vi "AD9959controlMR1_B1.vi"(9 "Enable Master Stepper":bool, 10 "Array":T2(array[cluster])=[{"Enable ASF?"=FALSE, "Channel Frequency (MHz)"=80.0, "ASF"=0.185, "Enable Frequency Sweep"=FALSE, "Sweep Parameters"={"Start Frequency (MHz)"=80.5, "Stop Frequency (MHz)"=89.25, "Rising Step Size (MHz)"=0.04375, "Falling Step Size (MHz)"=0.0, "Falling Step Interval (ms)"=0.01, "Rising Step Interval (ms)"=1.0}, "Rising/Falling"=FALSE}, {"Enable ASF?"=TRUE, "Channel Frequency (MHz)"=110.0, "ASF"=0.185, "Enable Frequency Sweep"=FALSE, "Sweep Parameters"={"Start Frequency (MHz)"=70.0, "Stop Frequency (MHz)"=160.0, "Rising Step Size (MHz)"=0.0006, "Falling Step Size (MHz)"=0.0, "Falling Step Interval (ms)"=0.01, "Rising Step Interval (ms)"=1.0}, "Rising/Falling"=FALSE}, {"Enable ASF?"=FALSE, "Channel Frequency (MHz)"=80.0, "ASF"=0.1, "Enable Frequency Sweep"=FALSE, "Sweep Parameters"={"Start Frequency (MHz)"=80.5, "Stop Frequency (MHz)"=89.25, "Rising Step Size (MHz)"=0.04375, "Falling Step Size (MHz)"=0.0, "Falling Step Interval (ms)"=0.01, "Rising Step Interval (ms)"=1.0}, "Rising/Falling"=FALSE}, {"Enable ASF?"=TRUE, "Channel Frequency (MHz)"=80.0, "ASF"=0.1, "Enable Frequency Sweep"=FALSE, "Sweep Parameters"={"Start Frequency (MHz)"=40.0, "Stop Frequency (MHz)"=115.0, "Rising Step Size (MHz)"=0.0006, "Falling Step Size (MHz)"=0.0, "Falling Step Interval (ms)"=0.01, "Rising Step Interval (ms)"=1.0}, "Rising/Falling"=FALSE}] {"Sweep Parameters"."Rising Step Interval (ms)" min=0.0 max=2.55 step=0.01 format="%.4f"; "Sweep Parameters"."Stop Frequency (MHz)" min=0.0 max=400.0 step=1.0 format="%.6f"; "Sweep Parameters"."Start Frequency (MHz)" min=0.0 max=400.0 step=1.0 format="%.6f"; "Sweep Parameters"."Falling Step Interval (ms)" min=0.0 max=2.55 step=0.01 format="%.2f"; "Sweep Parameters"."Falling Step Size (MHz)" min=0.0 max=400.0 step=0.1 format="%.6f"; "Sweep Parameters"."Rising Step Size (MHz)" min=0.0 max=400.0 step=0.1 format="%.7f"; "ASF" min=0.0 max=1.0 step=0.001 format="%.3f"; "Channel Frequency (MHz)" min=0.0 max=400.0 step=1.0 format="%.6f"}, 11 "VISA Reference":refnum<visa-resource-name>="AD1") -> (2 "Duration array":T1(array[cluster]))   [LabVIEW 2016]
uses:
  <userlib>/configTool/configTool.llb/initConfigGlobal.vi
  <userlib>/configTool/configTool.llb/addProperty(DBL).vi
  <userlib>/configTool/configTool.llb/addProperty(BOOL).vi
  <userlib>/configTool/configTool.llb/saveConfigFile - Text.vi
  <userlib>/configTool/configTool.llb/closeConfig.vi
panel:
  out "Actual Channel Frequencies (MHz)":dbl[](array[numeric]) format="%#_10g"
  out "error out 2":errorcluster
  in  "config file path":path
  in  "Save Config File":bool=TRUE
  in  "Load Config File?":bool=TRUE
  out "System Clock (MHz)":u32
  in  "Multiplier":u32=5
  in  "Reference Clock (MHz)":u32=20
  # "70-160MHz sweep"
  # "40-115MHz sweep"
  # "AD1"
  # "Unused"
  # "AOM3 IntraAction 110 MHz\nProbe 1"
  # "AOM4 Isomet 80 MHz\nProbe 2"
  # "AOM3 Intraction 110 MHz\nCalibration tone"
  # "max 0.115"
  # "max 0.185"
  # "max 0.100"
  # "max 0.185"
  # "Channel 1"
  # "Channel 2"
  # "Channel 3"
  # "Channel 0"
  # "I/O"
  # "Clock"
  # "Profile Pins"
  # "P0 is cut\nP1 is cut\nP2 is cut\nP3 is cut"
  # "Power Down"
  # "Notes:\nMinimum Frequency Step is 0.0931 Hz.\nMinimum ASF Step is 0.001"
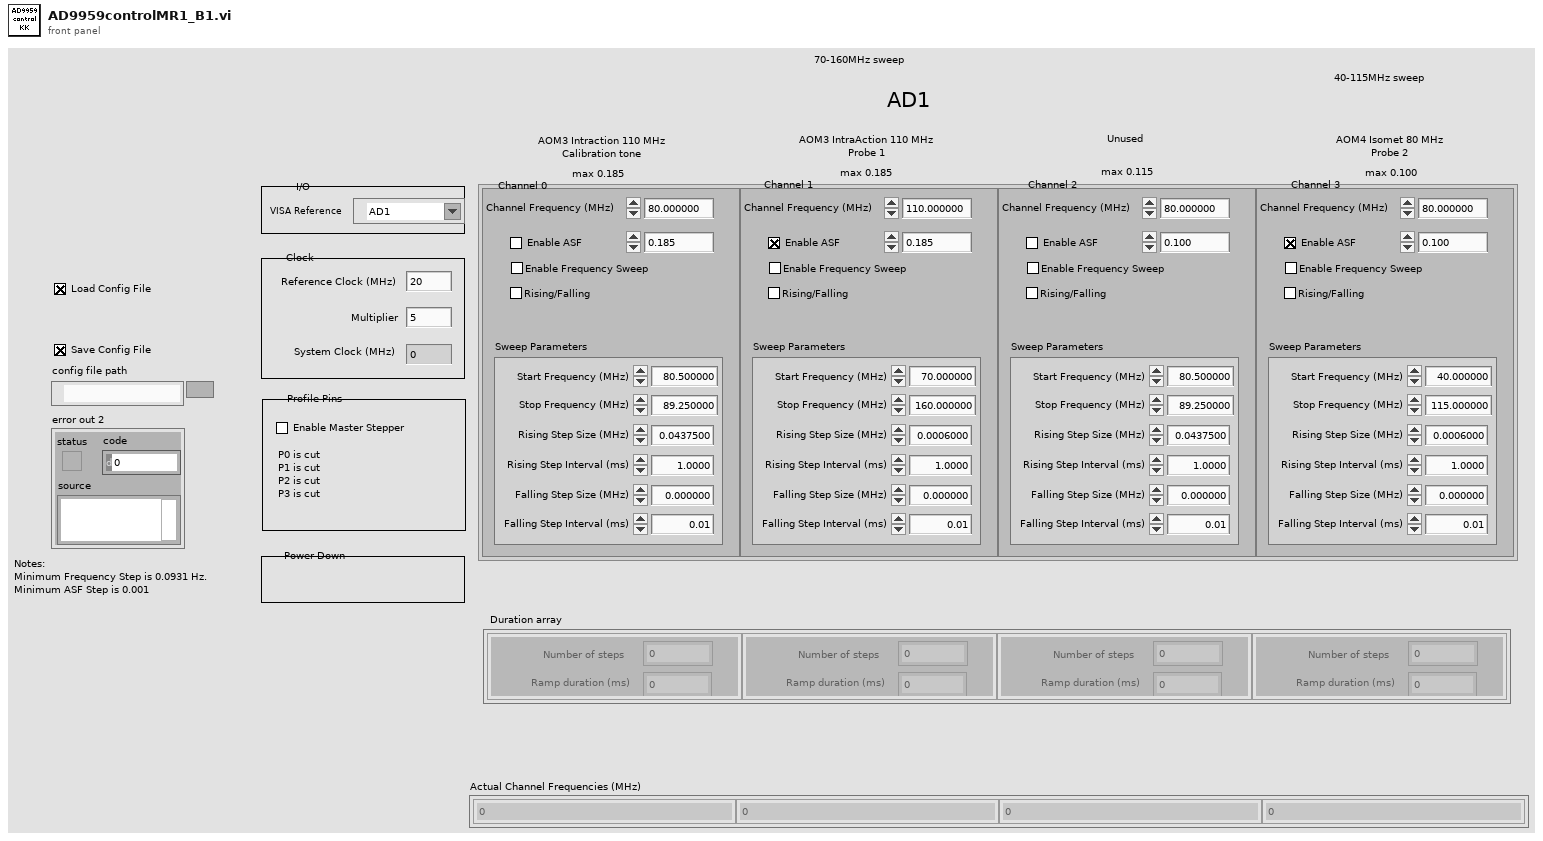
[diagram p1: front panel]
types:
  T1 = cluster{"Number of steps":dbl, "Ramp duration (ms)":dbl}[]
  T2 = cluster{"Enable ASF?":bool, "Channel Frequency (MHz)":dbl, "ASF":dbl, "Enable Frequency Sweep":bool, "Sweep Parameters":cluster{"Start Frequency (MHz)":dbl, "Stop Frequency (MHz)":dbl, "Rising Step Size (MHz)":dbl, "Falling Step Size (MHz)":dbl, "Falling Step Interval (ms)":dbl, "Rising Step Interval (ms)":dbl}, "Rising/Falling":bool}[]
  T3 = cluster{"Start Frequency (MHz)":dbl, "Stop Frequency (MHz)":dbl, "Rising Step Size (MHz)":dbl, "Falling Step Size (MHz)":dbl, "Falling Step Interval (ms)":dbl, "Rising Step Interval (ms)":dbl}[]
  T4 = cluster{"# of steps":dbl, "Ramp duration (ms)":dbl}[]
  T5 = cluster{"# of steps":dbl, "Ramp duration (ms)":dbl}
  T6 = cluster{"Start Frequency (MHz)":dbl, "Stop Frequency (MHz)":dbl, "Rising Step Size (MHz)":dbl, "Falling Step Size (MHz)":dbl, "Falling Step Interval (ms)":dbl, "Rising Step Interval (ms)":dbl}
  T7 = typedef "configRef.ctl" = refnum<vi>
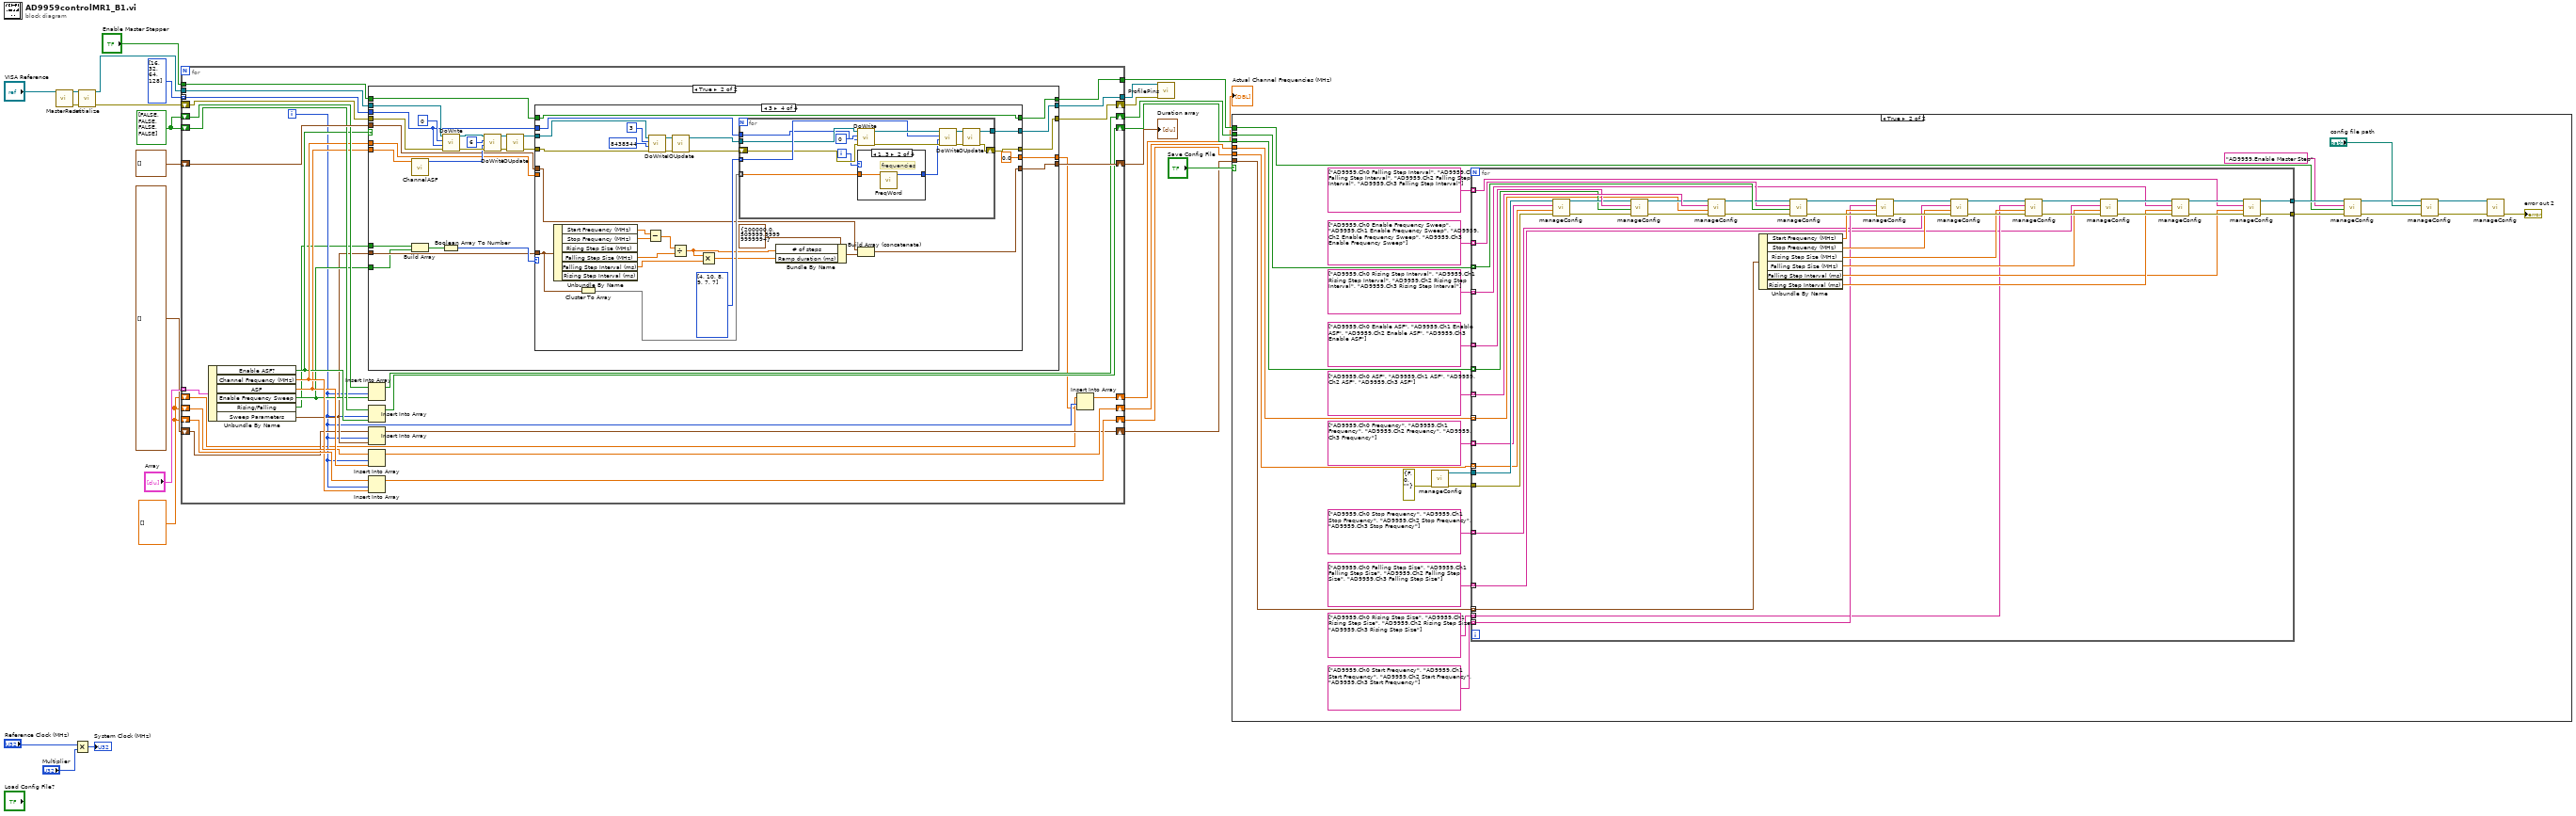
[diagram p0: block diagram]
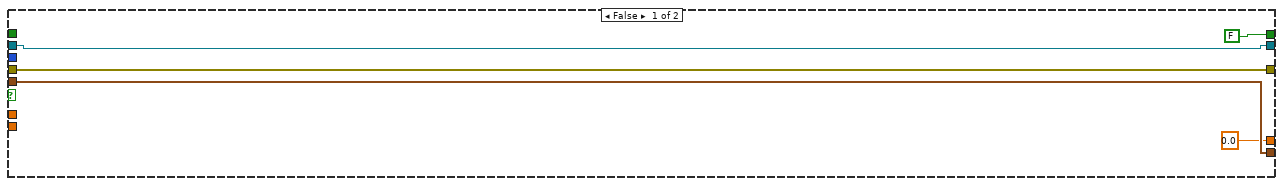
[diagram p3: hidden frame]
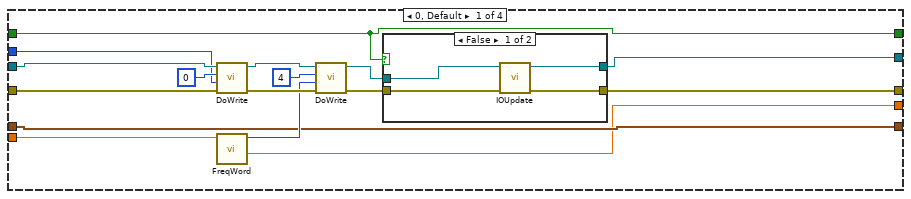
[diagram p4: hidden frame]
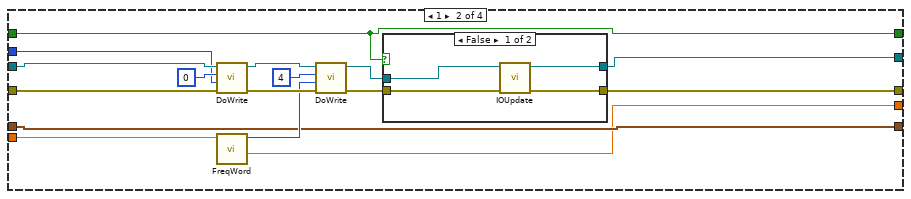
[diagram p6: hidden frame]
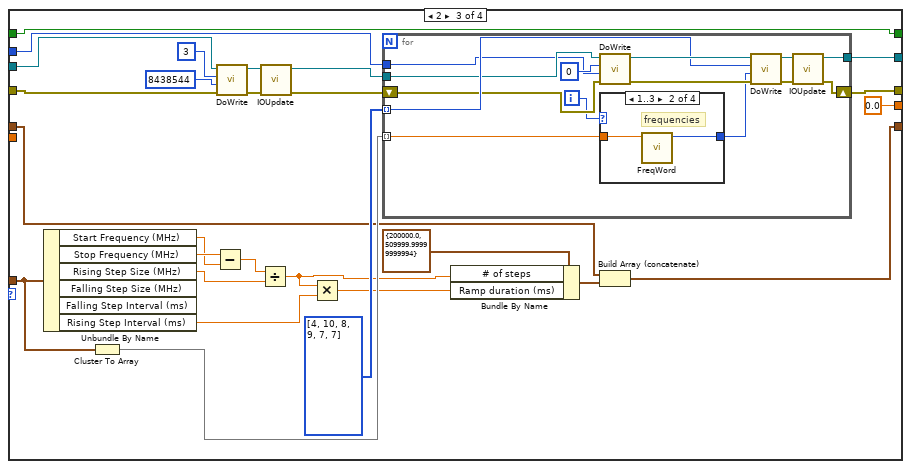
[diagram p8: hidden frame]
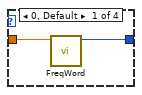
[diagram p9: hidden frame]
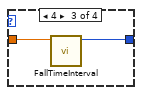
[diagram p10: hidden frame]
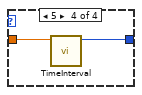
[diagram p11: hidden frame]
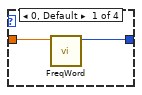
[diagram p12: hidden frame]
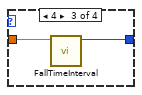
[diagram p13: hidden frame]
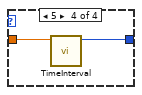
[diagram p14: hidden frame]
diagram:
  w2 = dbl[] [] ("array")
  w12 = bool[] [FALSE, FALSE, FALSE, FALSE] ("element")
  n1 = call "MasterReset.vi"("VISA Reference"="VISA Reference") -> ("error out"=w21:errorcluster, "dup VISA resource name"=w22:refnum<visa-resource-name>)  [unwired: 9 in]
  n2 = Multiply(x="Reference Clock (MHz)", y="Multiplier") -> (x*y=→"System Clock (MHz)":u32)
  n3 = call "Initialize.vi"("error in (no error)"=w21, "VISA Reference"=w22) -> ("error out"=w18:errorcluster, "dup VISA resource name"=w4:refnum<visa-resource-name>)  [unwired: 8 in]
  n4 = for {
    tunnel: "Array" -> [w56] mode=indexing
    tunnel: [w55] -> w3
    tunnel: w4 -> [w54]
    tunnel: u32[] [16, 32, 64, 128] ("Value 3") -> [w52] mode=indexing
    shift-right: [w51] -> w15
    shift-left: T4 [] -> [w50]
    shift-right: [w49] -> w19
    shift-left: w18 -> [w53]
    shift-right: [w47] -> w13
    shift-left: w12 -> [w48]
    shift-right: [w45] -> w11
    shift-left: w12 -> [w46]
    shift-right: [w42] -> w10
    shift-left: w2 -> [w44]
    shift-right: [w38] -> w8
    shift-left: w2 -> [w39]
    shift-right: [w34] -> w7
    shift-left: T3 [] ("array") -> [w35]
    tunnel: [w33] -> w6
    tunnel: "Enable Master Stepper" -> [w32]
    shift-right: [w29] -> w1
    shift-left: w2 -> [w30]
    i -> [w31]
    n5 = Unbundle By Name(w56) -> ("Enable ASF?"=w41:bool, "Channel Frequency (MHz)"=w43:dbl, "ASF"=w40:dbl, "Enable Frequency Sweep"=w37:bool, "Rising/Falling"=w27:bool, "Sweep Parameters"=w36:T6)
    n6 = case shown="True" w41 {
      tunnel: w54 -> [w61 w84]
      tunnel: w53 -> [w60 w85]
      tunnel: [w61 w76] -> w55
      tunnel: [w60 w75] -> w49
      tunnel: w40 -> [_ w74]
      tunnel: w37 -> [_ w63]
      tunnel: w43 -> [_ w73]
      tunnel: w36 -> [_ w65]
      tunnel: w52 -> [_ w72]
      tunnel: [w59 w69] -> w51
      tunnel: w50 -> [w59 w68]
      tunnel: [FALSE ("Enable Master Stepper") w67] -> w33
      tunnel: w32 -> [_ w66]
      tunnel: [0.0 ("Actual Frequency (MHz)") w64] -> w28
      tunnel: w27 -> [_ w62]
      frame False {
      }
      frame True {
        n7 = call "ChannelASF.vi"("ASF"=w74) -> ("ASF in hex"=w78:u32)  [unwired: 10 in]
        n8 = Build Array(w62, w63) -> (w70:bool[])
        n9 = Boolean Array To Number(Boolean array=w70) -> (number=w71:u32)
        n10 = call "DoWrite.vi"("error in (no error)"=w85, "Value"=w72, "Register Address"=0 ("Value 3"), "VISA Reference"=w84) -> ("error out"=w81:errorcluster, "dup VISA resource name"=w83:refnum<visa-resource-name>)  [unwired: 6 in]
        n11 = call "DoWrite.vi"("error in (no error)"=w81, "Value"=w78, "Register Address"=u32 6 ("Register Address 4"), "VISA Reference"=w83) -> ("error out"=w79:errorcluster, "dup VISA resource name"=w82:refnum<visa-resource-name>)  [unwired: 6 in]
        n12 = call "IOUpdate.vi"("error in (no error)"=w79, "VISA Reference"=w82) -> ("error out"=w86:errorcluster, "dup VISA resource name"=w87:refnum<visa-resource-name>)  [unwired: 8 in]
        n13 = case shown="3" w71 {
          tunnel: w86 -> [w96 w118 w155 w204]
          tunnel: w87 -> [w103 w125 w156 w205]
          tunnel: [w94 w116 w148 w197] -> w76
          tunnel: [w93 w115 w147 w196] -> w75
          tunnel: w73 -> [w92 w114 _ _]
          tunnel: w65 -> [_ _ w145 w194]
          tunnel: w72 -> [w91 w113 w146 w195]
          tunnel: [w90 w112 w134 w187] -> w69
          tunnel: w68 -> [w90 w112 w137 w190]
          tunnel: [w89 w111 w133 w186] -> w67
          tunnel: w66 -> [w89 w111 w133 w186]
          tunnel: [w88 w110 0.0 ("Actual Frequency (MHz)") 0.0 ("Actual Frequency (MHz)")] -> w64
          frame 0, Default {
            n14 = call "DoWrite.vi"("error in (no error)"=w96, "Value"=w91, "Register Address"=0 ("Value 3"), "VISA Reference"=w103) -> ("error out"=w102:errorcluster, "dup VISA resource name"=w101:refnum<visa-resource-name>)  [unwired: 6 in]
            n15 = call "FreqWord.vi"("Channel Frequency (MHz)"=w92) -> ("Actual Frequency (MHz)"=w88:dbl, "Frequency Tuning Word"=w97:u32)  [unwired: 9 in]
            n16 = call "DoWrite.vi"("error in (no error)"=w102, "Value"=w97, "Register Address"=u32 4 ("Register Address 2"), "VISA Reference"=w101) -> ("error out"=w99:errorcluster, "dup VISA resource name"=w100:refnum<visa-resource-name>)  [unwired: 6 in]
            n17 = case shown="False" w89 {
              tunnel: w100 -> [w107 w109]
              tunnel: w99 -> [w106 w108]
              tunnel: [w105 w109] -> w94
              tunnel: [w104 w108] -> w93
              frame False {
                n18 = call "IOUpdate.vi"("error in (no error)"=w106, "VISA Reference"=w107) -> ("error out"=w104:errorcluster, "dup VISA resource name"=w105:refnum<visa-resource-name>)  [unwired: 8 in]
              }
              frame True {
              }
            }
          }
          frame 1 {
            n19 = call "DoWrite.vi"("error in (no error)"=w118, "Value"=w113, "Register Address"=0 ("Value 3"), "VISA Reference"=w125) -> ("error out"=w124:errorcluster, "dup VISA resource name"=w123:refnum<visa-resource-name>)  [unwired: 6 in]
            n20 = call "FreqWord.vi"("Channel Frequency (MHz)"=w114) -> ("Actual Frequency (MHz)"=w110:dbl, "Frequency Tuning Word"=w119:u32)  [unwired: 9 in]
            n21 = call "DoWrite.vi"("error in (no error)"=w124, "Value"=w119, "Register Address"=u32 4 ("Register Address 2"), "VISA Reference"=w123) -> ("error out"=w121:errorcluster, "dup VISA resource name"=w122:refnum<visa-resource-name>)  [unwired: 6 in]
            n22 = case shown="False" w111 {
              tunnel: w122 -> [w129 w131]
              tunnel: w121 -> [w128 w130]
              tunnel: [w127 w131] -> w116
              tunnel: [w126 w130] -> w115
              frame False {
                n23 = call "IOUpdate.vi"("error in (no error)"=w128, "VISA Reference"=w129) -> ("error out"=w126:errorcluster, "dup VISA resource name"=w127:refnum<visa-resource-name>)  [unwired: 8 in]
              }
              frame True {
              }
            }
          }
          frame 2 {
            n24 = Unbundle By Name(w145) -> ("Start Frequency (MHz)"=w143:dbl, "Stop Frequency (MHz)"=w144:dbl, "Rising Step Size (MHz)"=w142:dbl, "Rising Step Interval (ms)"=w141:dbl)  [unwired: 2 out]
            n25 = Cluster To Array(cluster=w145) -> (array=w151:dbl[])
            n26 = Subtract(x=w144, y=w143) -> (x-y=w140:dbl)
            n27 = call "DoWrite.vi"("error in (no error)"=w155, "Value"=8438544 ("Value 3"), "Register Address"=3 ("Value 3"), "VISA Reference"=w156) -> ("error out"=w158:errorcluster, "dup VISA resource name"=w157:refnum<visa-resource-name>)  [unwired: 6 in]
            n28 = Divide(x=w140, y=w142) -> (x/y=w136:dbl)
            n29 = call "IOUpdate.vi"("error in (no error)"=w158, "VISA Reference"=w157) -> ("error out"=w150:errorcluster, "dup VISA resource name"=w149:refnum<visa-resource-name>)  [unwired: 8 in]
            n30 = Multiply(x=w136, y=w141) -> (x*y=w135:dbl)
            n31 = for {
              tunnel: i32[] [4, 10, 8, 9, 7, 7] -> [w168] mode=indexing
              shift-right: [w167] -> w147
              shift-left: w150 -> [w166]
              tunnel: w149 -> [w165]
              tunnel: [w160] -> w148
              tunnel: w151 -> [w162] mode=indexing
              tunnel: w146 -> [w159]
              i -> [w163]
              n32 = call "DoWrite.vi"("error in (no error)"=w166, "Value"=w159, "Register Address"=0 ("Value 3"), "VISA Reference"=w165) -> ("error out"=w169:errorcluster, "dup VISA resource name"=w170:refnum<visa-resource-name>)  [unwired: 6 in]
              n33 = case shown="1..3" w163 {
                tunnel: w162 -> [w174 w176 w178 w180]
                tunnel: [w173 w175 w177 w179] -> w161
                frame 0, Default {
                  n34 = call "FreqWord.vi"("Channel Frequency (MHz)"=w174) -> ("Frequency Tuning Word"=w173:u32)  [unwired: 9 in, 1 out]
                }
                frame 1..3 {
                  # "frequencies"
                  n35 = call "FreqWord.vi"("Channel Frequency (MHz)"=w176) -> ("Frequency Tuning Word"=w175:u32)  [unwired: 9 in, 1 out]
                }
                frame 4 {
                  n36 = call "FallTimeInterval.vi"("Fall Time Interval"=w178) -> ("Time interval in Hex"=w177:u32)  [unwired: 10 in]
                }
                frame 5 {
                  n37 = call "TimeInterval.vi"("Time Interval"=w180) -> ("Time interval in Hex"=w179:u32)  [unwired: 10 in]
                }
              }
              n38 = call "DoWrite.vi"("error in (no error)"=w169, "Value"=w161, "Register Address"=w168, "VISA Reference"=w170) -> ("error out"=w171:errorcluster, "dup VISA resource name"=w172:refnum<visa-resource-name>)  [unwired: 6 in]
              n39 = call "IOUpdate.vi"("error in (no error)"=w171, "VISA Reference"=w172) -> ("error out"=w167:errorcluster, "dup VISA resource name"=w160:refnum<visa-resource-name>)  [unwired: 8 in]
            }
            n40 = Bundle By Name(cluster=T5 {"# of steps"=200000.0, "Ramp duration (ms)"=509999.99999999994} ("Duration Cluster"), "# of steps"=w136, "Ramp duration (ms)"=w135) -> (w139:T5)
            n41 = Build Array (concatenate)(w137, w139) -> (w134:T4)
          }
          frame 3 {
            n42 = Unbundle By Name(w194) -> ("Start Frequency (MHz)"=w182:dbl, "Stop Frequency (MHz)"=w181:dbl, "Falling Step Size (MHz)"=w184:dbl, "Falling Step Interval (ms)"=w183:dbl)  [unwired: 2 out]
            n43 = Cluster To Array(cluster=w194) -> (array=w200:dbl[])
            n44 = Subtract(x=w182, y=w181) -> (x-y=w193:dbl)
            n45 = call "DoWrite.vi"("error in (no error)"=w204, "Value"=8438544 ("Value 3"), "Register Address"=3 ("Value 3"), "VISA Reference"=w205) -> ("error out"=w207:errorcluster, "dup VISA resource name"=w206:refnum<visa-resource-name>)  [unwired: 6 in]
            n46 = Divide(x=w193, y=w184) -> (x/y=w189:dbl)
            n47 = call "IOUpdate.vi"("error in (no error)"=w207, "VISA Reference"=w206) -> ("error out"=w199:errorcluster, "dup VISA resource name"=w198:refnum<visa-resource-name>)  [unwired: 8 in]
            n48 = Multiply(x=w189, y=w183) -> (x*y=w188:dbl)
            n49 = for {
              tunnel: i32[] [4, 10, 8, 9, 7, 7] -> [w217] mode=indexing
              shift-right: [w216] -> w196
              shift-left: w199 -> [w215]
              tunnel: w198 -> [w214]
              tunnel: [w209] -> w197
              tunnel: w200 -> [w211] mode=indexing
              tunnel: w195 -> [w208]
              i -> [w212]
              n50 = call "DoWrite.vi"("error in (no error)"=w215, "Value"=w208, "Register Address"=0 ("Value 3"), "VISA Reference"=w214) -> ("error out"=w218:errorcluster, "dup VISA resource name"=w219:refnum<visa-resource-name>)  [unwired: 6 in]
              n51 = case shown="1..3" w212 {
                tunnel: w211 -> [w223 w225 w227 w229]
                tunnel: [w222 w224 w226 w228] -> w210
                frame 0, Default {
                  n52 = call "FreqWord.vi"("Channel Frequency (MHz)"=w223) -> ("Frequency Tuning Word"=w222:u32)  [unwired: 9 in, 1 out]
                }
                frame 1..3 {
                  # "frequencies"
                  n53 = call "FreqWord.vi"("Channel Frequency (MHz)"=w225) -> ("Frequency Tuning Word"=w224:u32)  [unwired: 9 in, 1 out]
                }
                frame 4 {
                  n54 = call "FallTimeInterval.vi"("Fall Time Interval"=w227) -> ("Time interval in Hex"=w226:u32)  [unwired: 10 in]
                }
                frame 5 {
                  n55 = call "TimeInterval.vi"("Time Interval"=w229) -> ("Time interval in Hex"=w228:u32)  [unwired: 10 in]
                }
              }
              n56 = call "DoWrite.vi"("error in (no error)"=w218, "Value"=w210, "Register Address"=w217, "VISA Reference"=w219) -> ("error out"=w220:errorcluster, "dup VISA resource name"=w221:refnum<visa-resource-name>)  [unwired: 6 in]
              n57 = call "IOUpdate.vi"("error in (no error)"=w220, "VISA Reference"=w221) -> ("error out"=w216:errorcluster, "dup VISA resource name"=w209:refnum<visa-resource-name>)  [unwired: 8 in]
            }
            n58 = Bundle By Name(cluster=T5 {"# of steps"=200000.0, "Ramp duration (ms)"=509999.99999999994} ("Duration Cluster"), "# of steps"=w189, "Ramp duration (ms)"=w188) -> (w192:T5)
            n59 = Build Array (concatenate)(w190, w192) -> (w187:T4)
          }
        }
      }
    }
    n60 = Insert Into Array(array=w46, index=w31, new element=w37) -> (w45:bool[])
    n61 = Insert Into Array(array=w48, index=w31, new element=w41) -> (w47:bool[])
    n62 = Insert Into Array(array=w35, index=w31, new element=w36) -> (w34:T3)
    n63 = Insert Into Array(array=w39, index=w31, new element=w40) -> (w38:dbl[])
    n64 = Insert Into Array(array=w44, index=w31, new element=w43) -> (w42:dbl[])
    n65 = Insert Into Array(array=w30, index=w31, new element=w28) -> (w29:dbl[])
  }
  "Duration array" <- w15
  "Actual Channel Frequencies (MHz)" <- w1
  n66 = call "ProfilePins.vi"("error in (no error)"=w19, "VISA Reference"=w3) -> ()  [unwired: 8 in, 2 out]
  n67 = case shown="True" "Save Config File" {
    tunnel: w13 -> [_ w250]
    tunnel: w11 -> [_ w248]
    tunnel: w10 -> [_ w245]
    tunnel: w8 -> [_ w244]
    tunnel: w7 -> [_ w242]
    tunnel: w6 -> [_ w230]
    frame False {
    }
    frame True {
      n68 = call-poly <userlib>:"manageConfig.vi"("error in (no error)"=errorcluster {"status"=FALSE, "code"=0, "source"=""}) -> ("error out"=w247:errorcluster, "config ref out"=w252:T7)  [unwired: 9 in]
      n69 = for {
        tunnel: w252 -> [w295]
        tunnel: [w259] -> w235
        tunnel: string[] ["AD9959.Ch0 ASF", "AD9959.Ch1 ASF", "AD9959.Ch2 ASF", "AD9959.Ch3 ASF"] ("property path") -> [w300] mode=indexing
        tunnel: w250 -> [w290] mode=indexing
        tunnel: [w258] -> w234
        tunnel: string[] ["AD9959.Ch0 Enable ASF", "AD9959.Ch1 Enable ASF", "AD9959.Ch2 Enable ASF", "AD9959.Ch3 Enable ASF"] ("property path") -> [w298] mode=indexing
        tunnel: w248 -> [w287] mode=indexing
        tunnel: w247 -> [w293]
        tunnel: string[] ["AD9959.Ch0 Frequency", "AD9959.Ch1 Frequency", "AD9959.Ch2 Frequency", "AD9959.Ch3 Frequency"] ("property path") -> [w292] mode=indexing
        tunnel: w245 -> [w291] mode=indexing
        tunnel: w244 -> [w289] mode=indexing
        tunnel: string[] ["AD9959.Ch0 Enable Frequency Sweep", "AD9959.Ch1 Enable Frequency Sweep", "AD9959.Ch2 Enable Frequency Sweep", "AD9959.Ch3 Enable Frequency Sweep"] ("property path") -> [w285] mode=indexing
        tunnel: w242 -> [w284] mode=indexing
        tunnel: string[] ["AD9959.Ch0 Start Frequency", "AD9959.Ch1 Start Frequency", "AD9959.Ch2 Start Frequency", "AD9959.Ch3 Start Frequency"] ("property path") -> [w265] mode=indexing
        tunnel: string[] ["AD9959.Ch0 Stop Frequency", "AD9959.Ch1 Stop Frequency", "AD9959.Ch2 Stop Frequency", "AD9959.Ch3 Stop Frequency"] ("property path") -> [w264] mode=indexing
        tunnel: string[] ["AD9959.Ch0 Rising Step Size", "AD9959.Ch1 Rising Step Size", "AD9959.Ch2 Rising Step Size", "AD9959.Ch3 Rising Step Size"] ("property path") -> [w263] mode=indexing
        tunnel: string[] ["AD9959.Ch0 Falling Step Size", "AD9959.Ch1 Falling Step Size", "AD9959.Ch2 Falling Step Size", "AD9959.Ch3 Falling Step Size"] ("property path") -> [w262] mode=indexing
        tunnel: string[] ["AD9959.Ch0 Rising Step Interval", "AD9959.Ch1 Rising Step Interval", "AD9959.Ch2 Rising Step Interval", "AD9959.Ch3 Rising Step Interval"] ("property path") -> [w261] mode=indexing
        tunnel: string[] ["AD9959.Ch0 Falling Step Interval", "AD9959.Ch1 Falling Step Interval", "AD9959.Ch2 Falling Step Interval", "AD9959.Ch3 Falling Step Interval"] ("property path") -> [w260] mode=indexing
        n70 = call-poly <userlib>:"manageConfig.vi"("error in (no error)"=w293, "value"=w291, "property path"=w292, "config ref"=w295) -> ("error out"=w294:errorcluster, "config ref out"=w296:T7)  [unwired: 6 in]
        n71 = call-poly <userlib>:"manageConfig.vi"("error in (no error)"=w294, "value"=w290, "property path"=w298, "config ref"=w296) -> ("error out"=w297:errorcluster, "config ref out"=w299:T7)  [unwired: 6 in]
        n72 = call-poly <userlib>:"manageConfig.vi"("error in (no error)"=w297, "value"=w289, "property path"=w300, "config ref"=w299) -> ("error out"=w288:errorcluster, "config ref out"=w286:T7)  [unwired: 6 in]
        n73 = Unbundle By Name(w284) -> ("Start Frequency (MHz)"=w271:dbl, "Stop Frequency (MHz)"=w270:dbl, "Rising Step Size (MHz)"=w269:dbl, "Falling Step Size (MHz)"=w268:dbl, "Falling Step Interval (ms)"=w266:dbl, "Rising Step Interval (ms)"=w267:dbl)
        n74 = call-poly <userlib>:"manageConfig.vi"("error in (no error)"=w288, "value"=w287, "property path"=w285, "config ref"=w286) -> ("error out"=w272:errorcluster, "config ref out"=w273:T7)  [unwired: 6 in]
        n75 = call-poly <userlib>:"manageConfig.vi"("error in (no error)"=w272, "value"=w271, "property path"=w265, "config ref"=w273) -> ("error out"=w278:errorcluster, "config ref out"=w283:T7)  [unwired: 6 in]
        n76 = call-poly <userlib>:"manageConfig.vi"("error in (no error)"=w278, "value"=w270, "property path"=w264, "config ref"=w283) -> ("error out"=w277:errorcluster, "config ref out"=w282:T7)  [unwired: 6 in]
        n77 = call-poly <userlib>:"manageConfig.vi"("error in (no error)"=w277, "value"=w269, "property path"=w263, "config ref"=w282) -> ("error out"=w276:errorcluster, "config ref out"=w281:T7)  [unwired: 6 in]
        n78 = call-poly <userlib>:"manageConfig.vi"("error in (no error)"=w276, "value"=w268, "property path"=w262, "config ref"=w281) -> ("error out"=w275:errorcluster, "config ref out"=w280:T7)  [unwired: 6 in]
        n79 = call-poly <userlib>:"manageConfig.vi"("error in (no error)"=w275, "value"=w267, "property path"=w261, "config ref"=w280) -> ("error out"=w274:errorcluster, "config ref out"=w279:T7)  [unwired: 6 in]
        n80 = call-poly <userlib>:"manageConfig.vi"("error in (no error)"=w274, "value"=w266, "property path"=w260, "config ref"=w279) -> ("error out"=w258:errorcluster, "config ref out"=w259:T7)  [unwired: 6 in]
      }
      n81 = call-poly <userlib>:"manageConfig.vi"("error in (no error)"=w234, "value"=w230, "property path"="AD9959.Enable Master Step", "config ref"=w235) -> ("error out"=w233:errorcluster, "config ref out"=w232:T7)  [unwired: 6 in]
      n82 = call-poly <userlib>:"manageConfig.vi"("error in"=w233, "config file path"="config file path", "config ref"=w232) -> ("error out"=w257:errorcluster, "config ref out"=w256:T7)  [unwired: 6 in, 1 out]
      n83 = call-poly <userlib>:"manageConfig.vi"("error in (no error)"=w257, "config ref"=w256) -> ("error out"=→"error out 2":errorcluster)  [unwired: 9 in]
    }
  }
